vi "MIT Data Translator.vi"() -> ()   [LabVIEW 2014]
panel:
  out "Bin 2":i16 format="%016b"
  out "Signed Dec":i16
  in  "Unsigned to Signed":u16
  out "Hex":u16 format="%x"
  out "Bin":u16 format="%016b"
  out "Dec":u16
  in  "Numeric":i16
  # "EE >>> MIT"
  # "MIT >> EE"
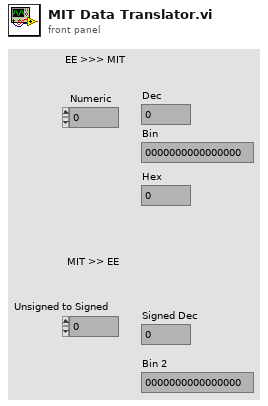
[diagram p1: front panel]
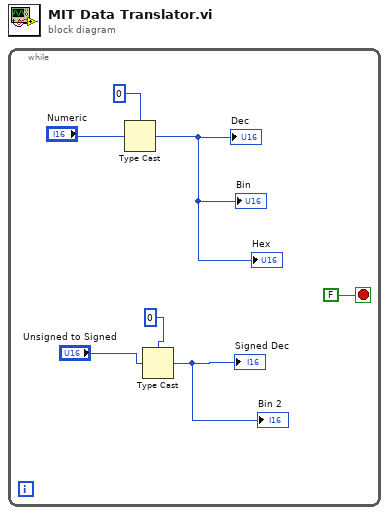
[diagram p0: block diagram]
diagram:
  n1 = while {
    stop <- FALSE stop-if-true
    n2 = Type Cast(type=u16 0, x="Numeric") -> (*(type *) &x=→"Dec" →"Bin" →"Hex":u16)
    n3 = Type Cast(type=i16 0, x="Unsigned to Signed") -> (*(type *) &x=→"Signed Dec" →"Bin 2":i16)
  }
